vi "DashboardGetProgramState.vi"(8 "Dashboard":refnum<k24>, 11 "error in":errorcluster) -> (0 "Response":cluster{"Message":string, "Succeed":bool}, 1 "State":i32(ring) items=["Stopped", "Playing", "Paused"], 2 "Name":string, 3 "error out":errorcluster)   [LabVIEW 2024, in "UnderAutomation.UniversalRobots.lvlib"]
uses:
  UnderAutomation.UniversalRobots.lvlib
  C:/Users/fg/Documents/UniversalRobots.vi/LabVIEW_2024/UnderAutomation.UniversalRobots/lib/UnderAutomation.UniversalRobots.dll
  lib/UnderAutomation.UniversalRobots.dll
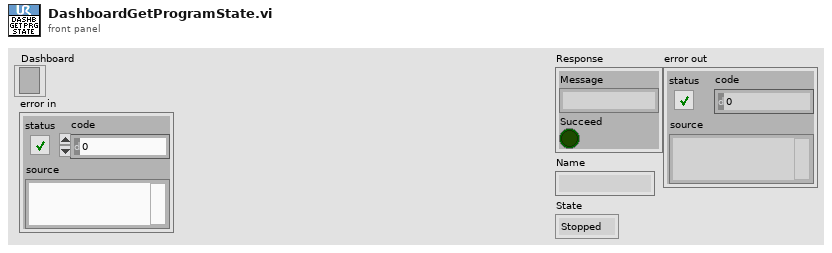
[diagram p1: front panel]
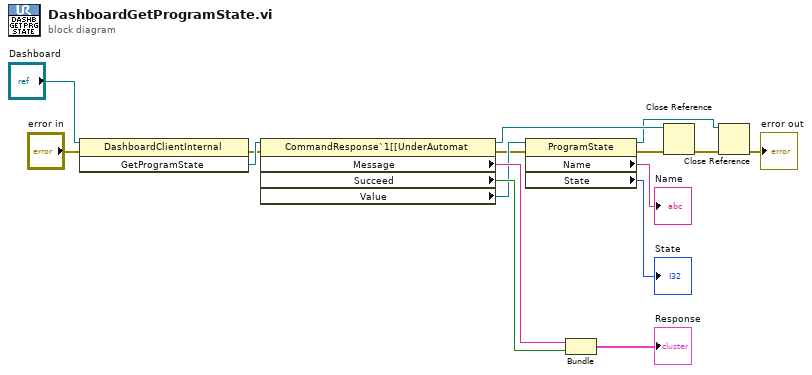
[diagram p0: block diagram]
diagram:
  n1 = invoke class="DashboardClientInternal" method="GetProgramState"(reference="Dashboard", error in="error in") -> (error out=w10:errorcluster, "GetProgramState"=w15:refnum<k24>)  [unwired: 1 in, 1 out]
  n2 = property class="CommandResponse`1[[UnderAutomat"(reference=w15, error in=w10) -> (reference out=w2:refnum<k24>, error out=w6:errorcluster, "Message"=w14:string, "Succeed"=w13:bool, "Value"=w9:refnum<k24>)
  n3 = property class="ProgramState"(reference=w9, error in=w6) -> (reference out=w1:refnum<k24>, error out=w5:errorcluster, "Name"=→"Name":string, "State"=→"State":i32)
  n4 = Bundle("Message"=w14, "Succeed"=w13) -> (→"Response":cluster{"Message":string, "Succeed":bool})  [unwired: 1 in]
  n5 = Close Reference(reference=w2, error in (no error)=w5) -> (error out=w4:errorcluster)
  n6 = Close Reference(reference=w1, error in (no error)=w4) -> (error out=→"error out":errorcluster)
